vi "Rebuild_Traceability.vi"() -> ()   [LabVIEW 2020]
doc: "Fonction :\n\nCe modèle peut être intégré très facilement à un subpannel à l'aide des fonctions de la palette Code Template >> Dynamic VI and Subpanel de la VIBOX"
uses:
  <vilib>/Utility/NIReport.llb/Report Type.ctl
  <vilib>/Utility/NIReport.llb/Append Text Table to Report (wrap).vi
  <vilib>/DataGrid for LabVIEW/source/DataGridView/DataGridView.lvclass
  C:/Program Files (x86)/National Instruments/LabVIEW 2020/examples/DataGrid for LabVIEW/DataGrid.lvlib
  <vilib>/Utility/NIReport.llb/NI_report.lvclass
  <vilib>/Utility/NIReport.llb/NI_ReportGenerationCore.lvlib
  System.Windows.Forms
panel:
  out "data":string[][](array[string])
  in  "搜索按钮":bool
  in  "追溯码":string
  out "Stop<user event>":refnum<user-event>
  in  "物料":refnum<k24>(container)
  in  "导出":bool
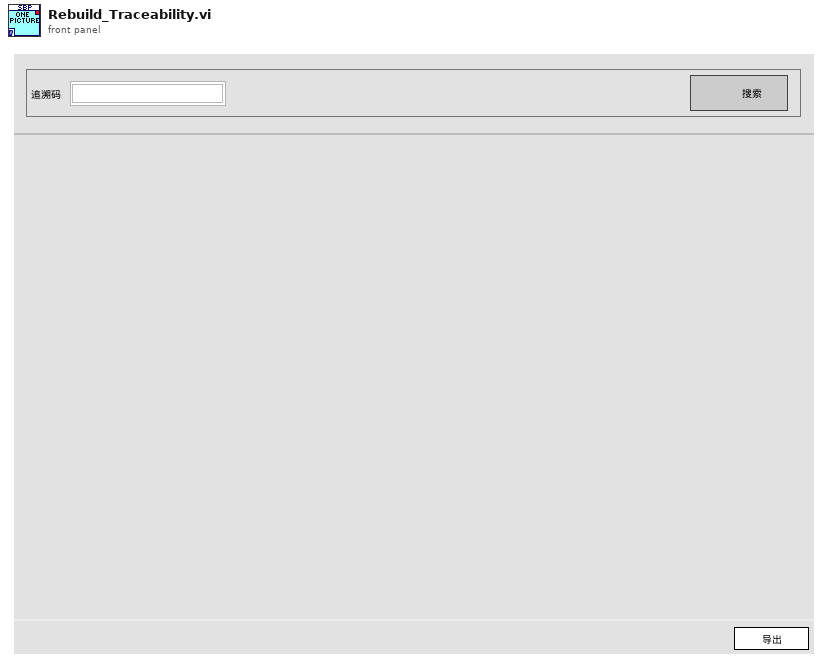
[diagram p1: front panel]
types:
  T1 = typedef "DataGrid.lvlib/GridColumn.lvclass/ColumnDefinition.ctl" = cluster{"name":string, "caption":string, "datatype":T2, "Params":string, "AutoSizeMode":i32, "FillWeight":sgl, "MinWidth":u32, "tooltip":string}
  T2 = typedef "DataGrid.lvlib/GridColumn.lvclass/ColumnType.ctl" = enum16{"string", "image", "check", "numeric", "timestamp", "button", "combo", "link"}
  T3 = typedef "NI_ReportGenerationCore.lvlib/Report Type.ctl" = enum16{"HTML", "Word", "Excel"}
  T4 = enum16{"maximized", "minimized", "normal", "no change"}
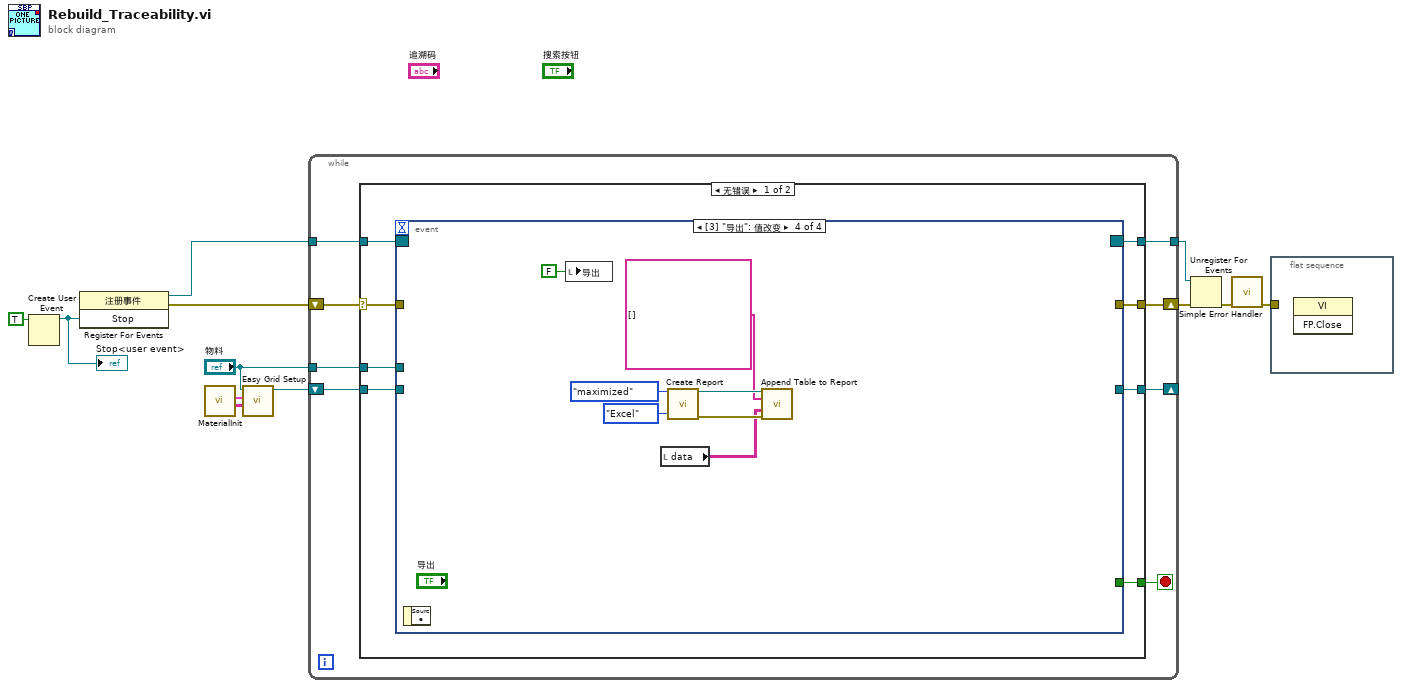
[diagram p0: block diagram]
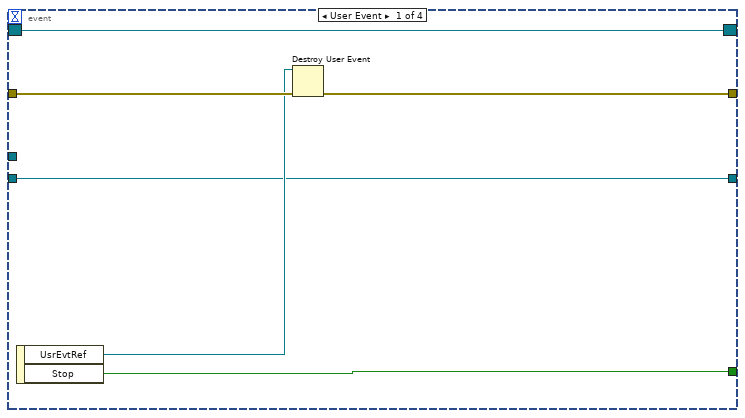
[diagram p2: hidden frame]
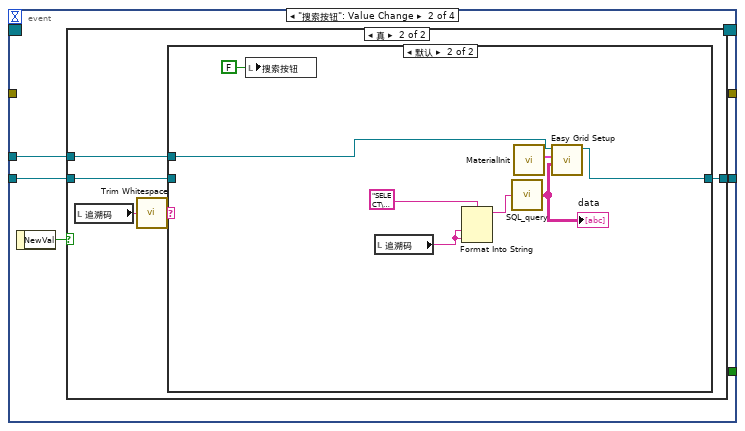
[diagram p3: hidden frame]
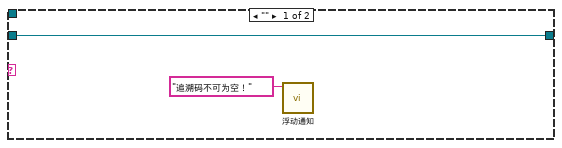
[diagram p5: hidden frame]
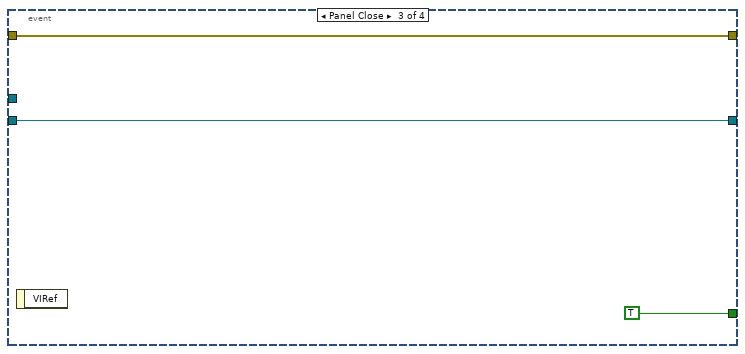
[diagram p6: hidden frame]
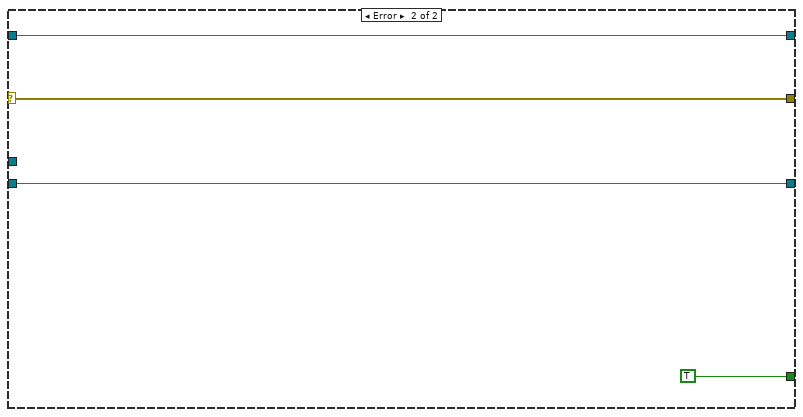
[diagram p7: hidden frame]
diagram:
  n1 = Create User Event(user event datatype=TRUE ("Stop")) -> (user event=w10:refnum<user-event>)  [unwired: 1 in, 1 out]
  "Stop<user event>" <- w10
  n2 = register-events(w10) -> (reference out=w9:refnum<event-registration>, error out=w5:errorcluster)  [unwired: 2 in]
  n3 = call "MaterialInit.vi"() -> ("DataSource Data"=w3:string[][], "ColumnSetup"=w4:T1[])  [unwired: 10 in]
  n4 = call <vilib>:"Easy Grid Setup.vi"("DataSource Data"=w3, "ColumnSetup"=w4, "DataGridView"="物料") -> ("DataGrid out"=w2:refnum<class "DataGridView.lvclass">)  [unwired: 5 in, 3 out]
  n5 = while {
    tunnel: w9 -> [w17]
    tunnel: [w16] -> w12
    shift-right: [w19] -> w8
    shift-left: w5 -> [w20]
    shift-right: [w14] -> _
    shift-left: w2 -> [w15]
    tunnel: "物料" -> [w13]
    stop <- w18 stop-if-true
    n6 = case shown="无错误" w20 {
      selector: w20 -> [w25 w67]
      tunnel: [w24 w67] -> w19
      tunnel: [w26 TRUE] -> w18
      tunnel: w17 -> [w27 w66]
      tunnel: [w28 w66] -> w16
      tunnel: w15 -> [w23 w65]
      tunnel: [w22 w65] -> w14
      tunnel: w13 -> [w21 _]
      frame No Error {
        n7 = event shown="[3] \"导出\": 值改变" {
          selector: w27 -> [w34 _ _ _]
          dyn-events: [w34 _ _ _] -> w28
          timeout: _ -> [_ _ _ _]
          tunnel: [w31 _ TRUE ("Stop") _] -> w26
          tunnel: w25 -> [w33 _ w56 _]
          tunnel: [w30 _ w56 _] -> w24
          tunnel: w23 -> [w29 w37 w55 _]
          tunnel: [w29 w36 w55 _] -> w22
          tunnel: w21 -> [_ w35 _ _]
          event User Event {
            n8 = event-data() -> ("UsrEvtRef"=w32:refnum<user-event>, "Stop"=w31:bool)  [unwired: 1 out]
            n9 = Destroy User Event(user event=w32, error in=w33) -> (error out=w30:errorcluster)
          }
          event "搜索按钮": Value Change {
            n10 = event-data() -> ("NewVal"=w38:bool)  [unwired: 1 out]
            n11 = case shown="真" w38 {
              tunnel: w37 -> [w39 w42]
              tunnel: [w39 w43] -> w36
              tunnel: w35 -> [_ w44]
              frame False {
              }
              frame True {
                n12 = local read "追溯码"() -> (w41:string)
                n13 = call <vilib>:"Trim Whitespace.vi"("string"=w41) -> ("trimmed string"=w40:string)  [unwired: 1 in]
                n14 = case shown="默认" w40 {
                  tunnel: w44 -> [_ w53]
                  tunnel: [w46 w52] -> w43
                  tunnel: w42 -> [w46 _]
                  frame "" {
                    n15 = call "浮动通知.vi"("通知内容"="追溯码不可为空！") -> ()  [unwired: 11 in]
                  }
                  frame Default {
                    n16 = local write "搜索按钮"(FALSE ("搜索按钮")) -> ()
                    n17 = local read "追溯码"() -> (w47:string)
                    n18 = Format Into String(format string="SELECT\ndbo.[不合格].[生产编号],\ndbo.[不合格].[产品型号],\ndbo.[不合格].[工位追溯码],\ndbo.[不合格].[总成追溯码],\ndbo.[不合格].[下线位置],\ndbo.[不合格].[重新上线位置],\ndbo.[不合格代码].[不合格代码]\n\nFROM\ndbo.[不合格]\nINNER JOIN dbo.[不合格代码] ON dbo.[不合格].[不合格代码] = dbo.[不合格代码].[不合格代码]\nWHERE\ndbo.[不合格].[总成追溯码] = N'%s' OR\ndbo.[不合格].[工位追溯码] = N'%s'", w47, w47) -> (resulting string=w49:string)  [unwired: 2 in, 1 out]
                    n19 = call "SQL_query.vi"("SQL query"=w49) -> ("data"=w50:string[][])  [unwired: 3 in, 1 out]
                    "data" <- w50
                    n20 = call "MaterialInit.vi"() -> ("ColumnSetup"=w51:T1[])  [unwired: 10 in, 1 out]
                    n21 = call <vilib>:"Easy Grid Setup.vi"("DataSource Data"=w50, "ColumnSetup"=w51, "DataGridView"=w53) -> ("DataGrid out"=w52:refnum<class "DataGridView.lvclass">)  [unwired: 5 in, 3 out]
                  }
                }
              }
            }
          }
          event Panel Close {
            n22 = event-data() -> ()  [unwired: 2 out]
          }
          event "导出": Value Change {
            n23 = event-data() -> ()  [unwired: 2 out]
            n24 = local write "导出"(FALSE ("导出")) -> ()
            n25 = local read "data"() -> (w59:string[][])
            n26 = call <vilib>:"Create Report.vi"("window state (normal)"=T4."maximized", "report type"=Report_Type."Excel") -> ("report out"=w61:refnum<class "NI_report.lvclass">, "error out"=w60:errorcluster)  [unwired: 12 in]
            n27 = call-poly <vilib>:"Append Table to Report.vi"("report in"=w61, "column headers"=string[] [], "text data"=w59, "error in (no error)"=w60) -> ()  [unwired: 8 in, 4 out]
          }
        }
      }
      frame Error {
      }
    }
  }
  n28 = Unregister For Events(event registration refnum=w12, error in=w8) -> (error out=w11:errorcluster)
  n29 = call <vilib>:"Simple Error Handler.vi"("error in (no error)"=w11) -> ("error out"=w6:errorcluster)  [unwired: 1 in, 7 out]
  n30 = flat-sequence {
    tunnel: w6 -> [_]
    frame #0 {
      n31 = invoke class="VI" method="FP.Close"() -> ()  [unwired: 3 in, 3 out]
    }
  }
